vi "Read 1Port 1Sampe U8.vi"(8 "error in (no error)":errorcluster, 10 "Port (Bank)":T1 items=["DIO1...8"=1, "DIO9...16"=2, "DIO17...24"=3, "DIO25...32"=4], 11 "MicroDAQ.lvlib:Digital Input.lvclass":refnum<class "Digital Input.lvclass">) -> (0 "error out":errorcluster, 2 "data":u8 format="%08b", 3 "MicroDAQ.lvlib:Digital Input.lvclass out":refnum<class "Digital Input.lvclass">)   [LabVIEW 2009, in "MicroDAQ.lvlib" / "Digital Input.lvclass"]
doc: "Reads a 1D Boolean array value from a digital input channel composed of a single port."
uses:
  <instrlib>/MicroDAQ/Channel/Digital Input/Digital Input.lvclass
  <instrlib>/MicroDAQ/Tools/Digital IO channels.ctl
  <instrlib>/MicroDAQ/MicroDAQ.lvlib
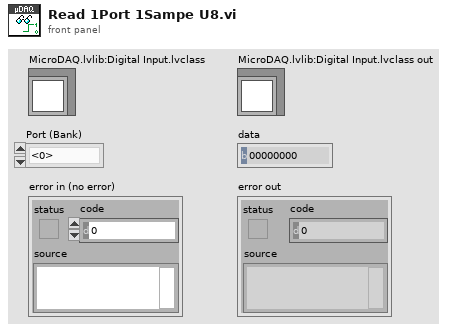
[diagram p1: front panel]
types:
  T1 = typedef "MicroDAQ.lvlib/Digital IO channels.ctl" = u8
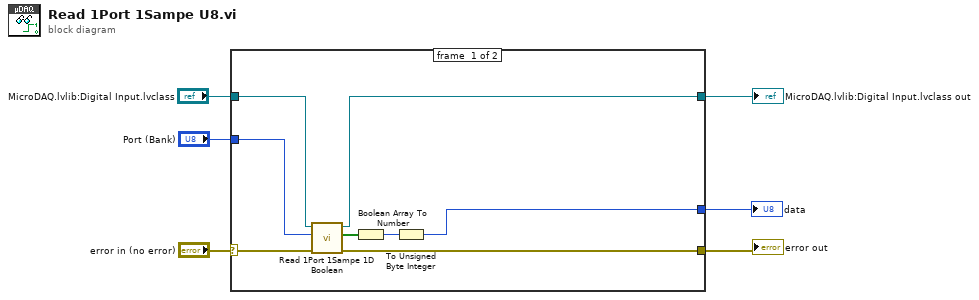
[diagram p0: block diagram]
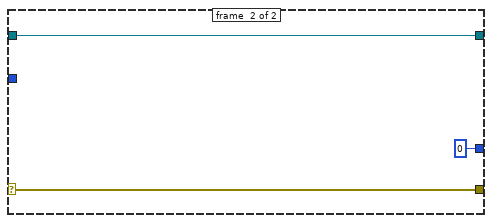
[diagram p2: hidden frame]
diagram:
  n1 = case shown="No Error" "error in (no error)" {
    selector: "error in (no error)" -> [w14 w16]
    tunnel: [w11 w16] -> w5
    tunnel: "MicroDAQ.lvlib:Digital Input.lvclass" -> [w13 w17]
    tunnel: [w7 w17] -> w3
    tunnel: "Port (Bank)" -> [w12 _]
    tunnel: [w8 u8 0] -> w1
    frame #0 {
      n2 = call <instrlib>:"Read 1Port 1Sampe 1D Boolean.vi"("error in (no error)"=w14, "Port (Bank)"=w12, "MicroDAQ.lvlib:Digital Input.lvclass"=w13) -> ("error out"=w11:errorcluster, "data"=w10:bool[], "MicroDAQ.lvlib:Digital Input.lvclass out"=w7:refnum<class "Digital Input.lvclass">)  [unwired: 6 in]
      n3 = Boolean Array To Number(Boolean array=w10) -> (number=w9:u32)
      n4 = To Unsigned Byte Integer(number=w9) -> (unsigned 8bit integer=w8:u8)
    }
    frame #1 {
    }
  }
  "error out" <- w5
  "MicroDAQ.lvlib:Digital Input.lvclass out" <- w3
  "data" <- w1
